vi "Find Newest CAN Logs.vi"(6 "# Queued":u16, 7 "CAN Sysdef Config":T1[](array[typedef]), 8 "error in (no error)":errorcluster) -> (0 "error out":errorcluster, 2 "Files To Transfer":string[](array[string]))   [LabVIEW 2010, in "CAN Log Transfer and Convert.lvlib"]
uses:
  CAN Log Transfer and Convert.lvlib
  CAN Sysdef Data.ctl
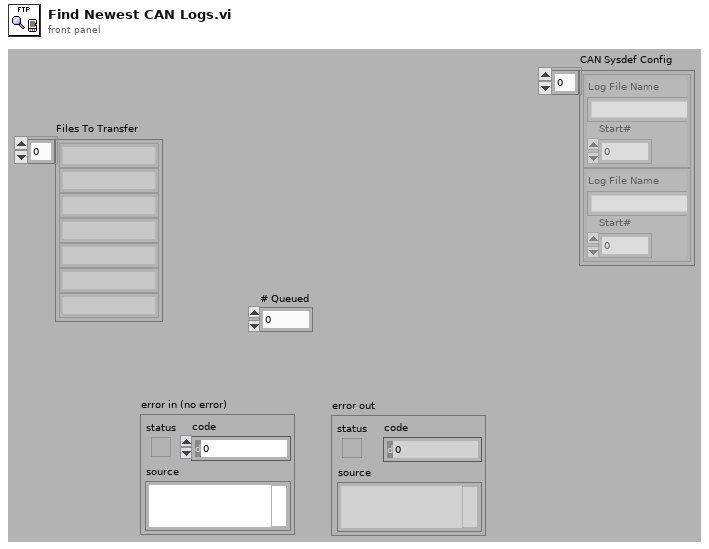
[diagram p1: front panel]
types:
  T1 = typedef "CAN Log Transfer and Convert.lvlib/CAN Sysdef Data.ctl" = cluster{"Log File Name":string, "Start#":u16}
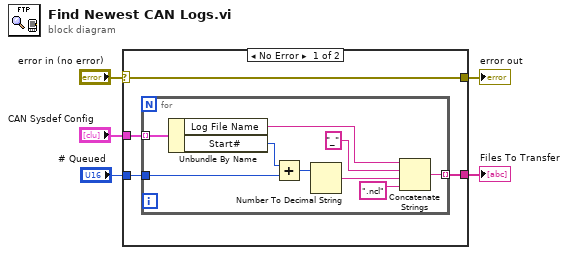
[diagram p0: block diagram]
diagram:
  n1 = case shown="No Error" "error in (no error)" {
    selector: "error in (no error)" -> [w6 w19]
    tunnel: "CAN Sysdef Config" -> [w9 _]
    tunnel: "# Queued" -> [w8 _]
    tunnel: [w7 _] -> w3
    tunnel: [w6 w19] -> w1
    frame No Error {
      n2 = for {
        tunnel: w9 -> [w18] mode=indexing
        tunnel: w8 -> [w15]
        tunnel: [w11] -> w7 mode=indexing
        n3 = Unbundle By Name(w18) -> ("Log File Name"=w17:string, "Start#"=w16:u16)
        n4 = Add(x=w16, y=w15) -> (x+y=w13:u16)
        n5 = Number To Decimal String(number=w13) -> (decimal integer string=w12:string)  [unwired: 1 in]
        n6 = Concatenate Strings(w17, "_" ("string"), w12, ".ncl" ("string")) -> (w11:string)
      }
    }
    frame Error {
    }
  }
  "Files To Transfer" <- w3
  "error out" <- w1
